vi "GetNumberTiles.vi"(5 "Digits":i32, 7 "AutoWidth? (f)":bool, 9 "Color":T1, 10 "score":i16) -> (3 "Tiles":u32[](array[numeric]))   [LabVIEW 2019, in "RT_Game.lvlib" / "Game.lvclass"]
uses:
  Game.lvclass
  Color.ctl
  RT_Game.lvlib
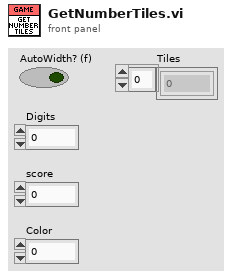
[diagram p1: front panel]
types:
  T1 = typedef "RT_Game.lvlib/Color.ctl" = fxp<+,3,3>
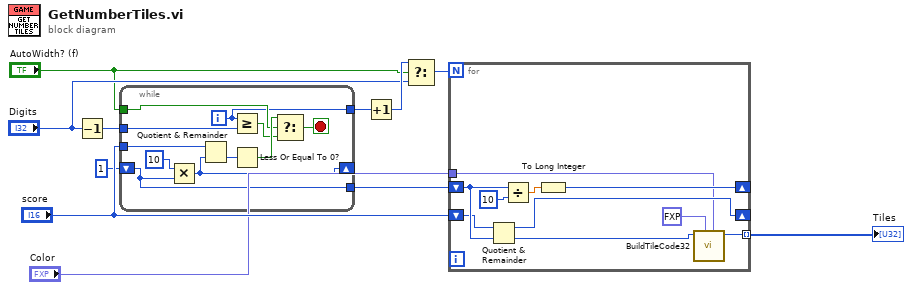
[diagram p0: block diagram]
diagram:
  n1 = Decrement(x="Digits") -> (x-1=w9:i32)
  n2 = while {
    shift-right: [w19] -> _
    shift-left: 1 -> [w20]
    tunnel: [w20] -> w4
    tunnel: "score" -> [w21]
    tunnel: "AutoWidth? (f)" -> [w14]
    tunnel: w9 -> [w15]
    tunnel: [w12] -> w10
    i -> [w12]
    stop <- w16 stop-if-true
    n3 = Multiply(x=10, y=w20) -> (x*y=w19:i32)
    n4 = Quotient & Remainder(x=w21, y=w19) -> (floor(x/y)=w18:i32)  [unwired: 1 out]
    n5 = Greater Or Equal?(x=w12, y=w15) -> (x >= y?=w13:bool)
    n6 = Less Or Equal To 0?(x=w18) -> (x <= 0?=w17:bool)
    n7 = Select(t=w17, s=w14, f=w13) -> (s? t:f=w16:bool)
  }
  n8 = Increment(x=w10) -> (x+1=w11:i32)
  n9 = Select(t=w11, s="AutoWidth? (f)", f="Digits") -> (s? t:f=w6:i32)
  n10 = for {
    N: w6 -> [_]
    shift-right: [w29] -> _
    shift-left: w4 -> [w32]
    shift-right: [w26] -> _
    shift-left: "score" -> [w27]
    tunnel: "Color" -> [w23]
    tunnel: [w28] -> w1 mode=indexing
    n11 = Quotient & Remainder(x=w27, y=w32) -> (x-y*floor(x/y)=w26:i32, floor(x/y)=w25:i32)
    n12 = Divide(x=w32, y=10) -> (x/y=w30:dbl)
    n13 = To Long Integer(number=w30) -> (32bit integer=w29:i32)
    n14 = call "BuildTileCode32.vi"("replacecolor"=w23, "color_to_replace"=fxp<+,3,3> 7.0, "Tilenumber"=w25) -> ("TileCode"=w28:u32)  [unwired: 8 in]
  }
  "Tiles" <- w1
